vi "Add Coin[].vi"(0 "1D Board":T1[](array[typedef]), 5 "Team Number":i32, 7 "Cell Index[]":i32[](array[numeric]), 11 "error in (no error)":errorcluster) -> (4 "Max Coin Wins":i32, 6 "Win?":bool, 8 "Cell Index":i32, 15 "error out":errorcluster)   [LabVIEW 2014]
uses:
  Typedefs/Board Cell.ctl
  Typedefs/Cell Occupancy.ctl
  Dragon Tamers.lvlib
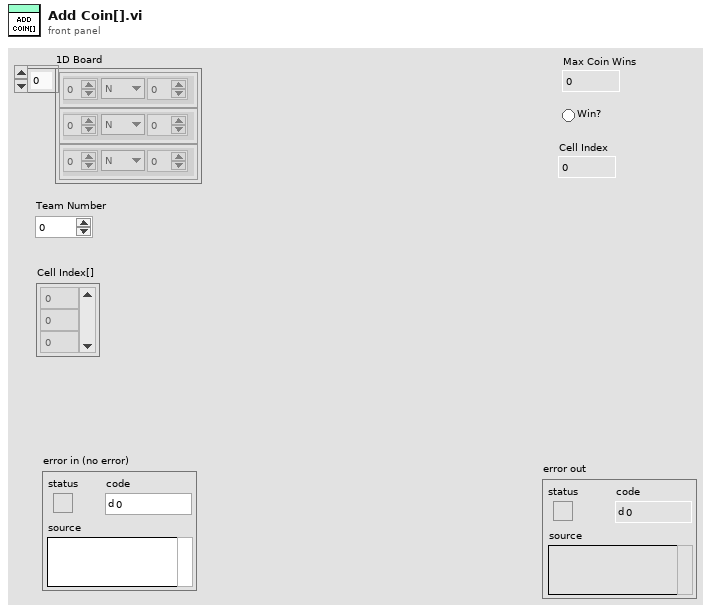
[diagram p1: front panel]
types:
  T1 = typedef "Dragon Tamers.lvlib/Board Cell.ctl" = cluster{"Team":i32, "Occu.":T2, "Count":i32}
  T2 = typedef "Dragon Tamers.lvlib/Cell Occupancy.ctl" = enum16{"N", "C", "K"}
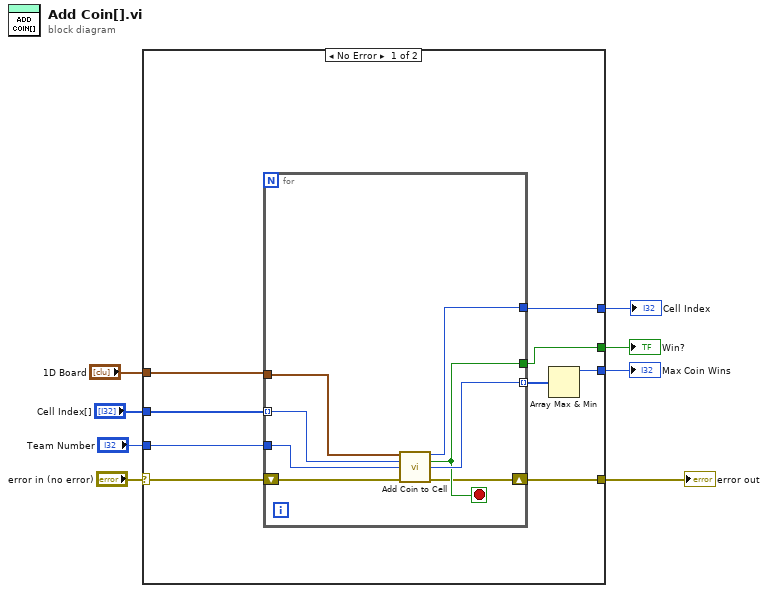
[diagram p0: block diagram]
diagram:
  n1 = case shown="No Error" "error in (no error)" {
    selector: "error in (no error)" -> [w17 w26]
    tunnel: [w16 w26] -> w7
    tunnel: "1D Board" -> [w15 _]
    tunnel: "Team Number" -> [w14 _]
    tunnel: "Cell Index[]" -> [w13 _]
    tunnel: [w11 _] -> w3
    tunnel: [w10 _] -> w2
    tunnel: [w9 _] -> w1
    frame No Error {
      n2 = for {
        tunnel: w15 -> [w25]
        shift-right: [w20] -> w16
        shift-left: w17 -> [w24]
        tunnel: [w23] -> w12 mode=indexing
        tunnel: [w22] -> w10
        tunnel: [w21] -> w9
        tunnel: w14 -> [w19]
        tunnel: w13 -> [w18] mode=indexing
        stop <- w22 stop-if-true
        n3 = call "Add Coin to Cell.vi"("1D Board Array"=w25, "Cell Index"=w18, "Team Number"=w19, "error in (no error)"=w24) -> ("Cell Index"=w21:i32, "Win?"=w22:bool, "Coins Won"=w23:i32, "error out"=w20:errorcluster)  [unwired: 7 in, 1 out]
      }
      n4 = Array Max & Min(array=w12) -> (max value=w11:i32)  [unwired: 3 out]
    }
    frame Error {
    }
  }
  "error out" <- w7
  "Max Coin Wins" <- w3
  "Win?" <- w2
  "Cell Index" <- w1
